vi "Set One Filter.vi"(8 "error in (no error)":errorcluster, 9 "Position (0:4)":i32, 10 "Filter Wheel (0:n-1)":i32, 11 "FW Arduino Control in":refnum<class "FW Arduino Control.lvclass">) -> (0 "error out":errorcluster, 1 "Actual Counts":i32, 2 "Curr Pos":i32, 3 "FW Arduino Control out":refnum<class "FW Arduino Control.lvclass">, 4 "Message":string, 6 "No Move?":bool)   [LabVIEW 2024, in "FW Arduino Control.lvclass"]
uses:
  FW Arduino Control.lvclass
  Filter Wheel Object/Filter Wheel.lvclass
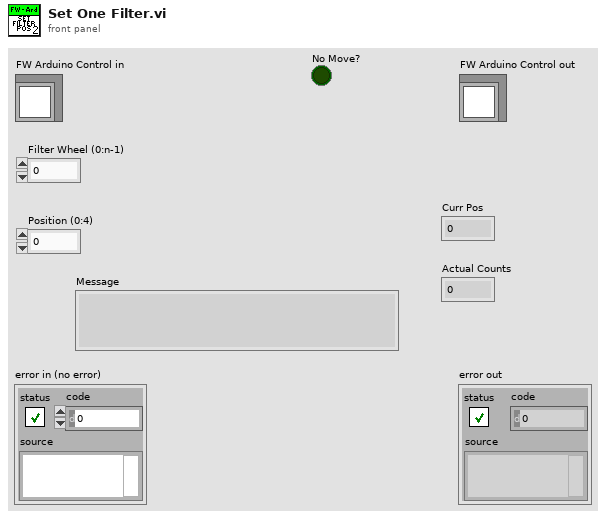
[diagram p1: front panel]
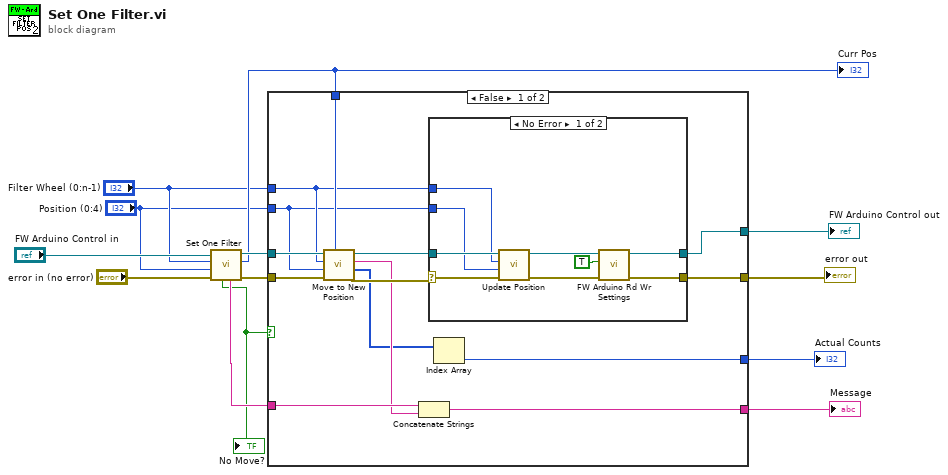
[diagram p0: block diagram]
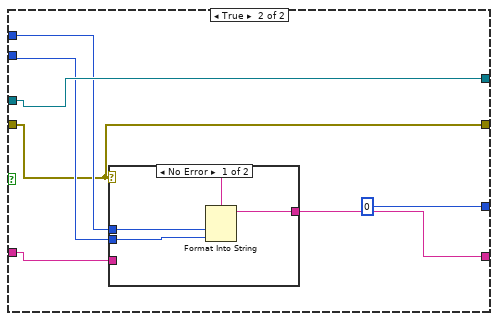
[diagram p3: hidden frame]
diagram:
  n1 = call-parent "Set One Filter.vi"("error in (no error)"="error in (no error)", "Position (0:4)"="Position (0:4)", "Filter Wheel (0:n-1)"="Filter Wheel (0:n-1)", "Filter Wheel in"="FW Arduino Control in") -> ("error out"=w11:errorcluster, "Curr Pos"=w9:i32, "Filter Wheel out"=w10:refnum<class "FW Arduino Control.lvclass">, "Message"=w8:string, "No Move?"=w1:bool)  [unwired: 2 in, 1 out]
  "Curr Pos" <- w9
  "No Move?" <- w1
  n2 = case shown="False" w1 {
    tunnel: w11 -> [w27 w39]
    tunnel: w10 -> [w26 w45]
    tunnel: w9 -> [w25 _]
    tunnel: w8 -> [w22 w40]
    tunnel: "Filter Wheel (0:n-1)" -> [w20 w43]
    tunnel: "Position (0:4)" -> [w19 w42]
    tunnel: [w18 w39] -> w5
    tunnel: [w17 w45] -> w4
    tunnel: [w16 w41] -> w3
    tunnel: [w14 0 ("Actual distance")] -> w2
    frame False {
      n3 = call "Move to New Position.vi"("Curr Filter"=w25, "error in (no error)"=w27, "Target Filter"=w19, "Filter Wheel (0:n-1)"=w20, "FW Arduino Control in"=w26) -> ("error out"=w24:errorcluster, "Actual Distance"=w15:i32[], "Log"=w21:string, "FW Arduino Control out"=w23:refnum<class "FW Arduino Control.lvclass">)  [unwired: 3 in]
      n4 = Concatenate Strings(w22, w21) -> (w16:string)
      n5 = case shown="No Error" w24 {
        selector: w24 -> [w34 w38]
        tunnel: w23 -> [w36 w37]
        tunnel: w20 -> [w35 _]
        tunnel: w19 -> [w33 _]
        tunnel: [w29 w38] -> w18
        tunnel: [w28 w37] -> w17
        frame No Error {
          n6 = call "Update Position.vi"("error in (no error)"=w34, "Position (0:4)"=w33, "Filter Wheel (0:n-1)"=w35, "Filter Wheel in"=w36) -> ("error out"=w30:errorcluster, "Filter Wheel out"=w31:refnum<class "FW Arduino Control.lvclass">)  [unwired: 6 in]
          n7 = call "FW Arduino Rd Wr Settings.vi"("error in (no error)"=w30, "Write? (F:Read)"=TRUE, "Settings"=w31) -> ("error out"=w29:errorcluster, "Settings"=w28:refnum<class "FW Arduino Control.lvclass">)  [unwired: 7 in]
        }
        frame Error {
        }
      }
      n8 = Index Array(array=w15) -> (element=w14:i32)  [unwired: 1 in]
    }
    frame True {
      n9 = case shown="No Error" w39 {
        tunnel: w43 -> [w48 _]
        tunnel: w42 -> [w47 _]
        tunnel: [w46 w50] -> w41
        tunnel: w40 -> [_ w50]
        frame No Error {
          n10 = Format Into String(format string="Wheel %d aready at filter %d", w48, w47) -> (resulting string=w46:string)  [unwired: 2 in, 1 out]
        }
        frame Error {
        }
      }
    }
  }
  "error out" <- w5
  "FW Arduino Control out" <- w4
  "Actual Counts" <- w2
  "Message" <- w3
